vi "Insert Vi by Node.vi"(8 "error in":errorcluster caption="错误输入（无错误）", 9 "dynamic VI*":refnum<vi>, 10 "Node*":refnum<data-value>, 11 "PanelRootNode 输入":refnum<class "PanelRootNode.lvclass"> caption="DNL_LabVIEW Object in") -> (0 "error out":errorcluster caption="错误输出", 3 "PanelRootNode 输出":refnum<class "PanelRootNode.lvclass"> caption="DNL_LabVIEW Object out")   [LabVIEW 2016, in "PanelRootNode.lvclass"]
uses:
  PanelRootNode.lvclass
  C:/Users/CL/Desktop/ZcDAQprj0811/ZcDAQprj/Modules/DAQ-Display/PanelSplitToolkit/PanelLinkNode/PanelLinkNode.lvclass
  PanelObject/PanelObject.lvclass
  PanelLinkNode/PanelLinkNode.lvclass/PanelLinkNode.ctl
  PanelDataNode/PanelDataNode.lvclass
  PanelLinkNode/PanelLinkNode.lvclass
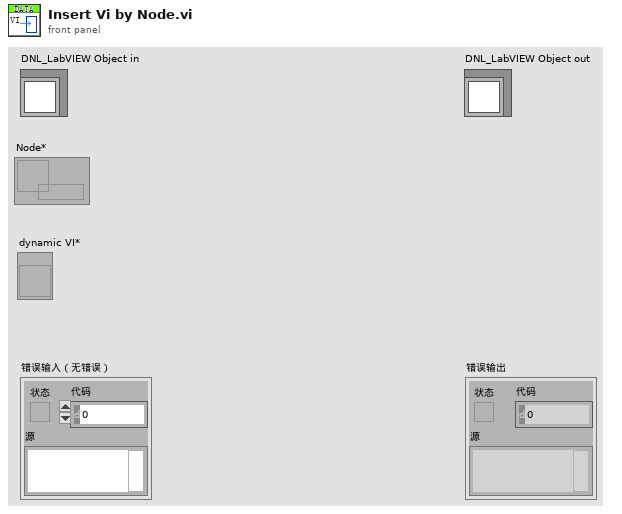
[diagram p1: front panel]
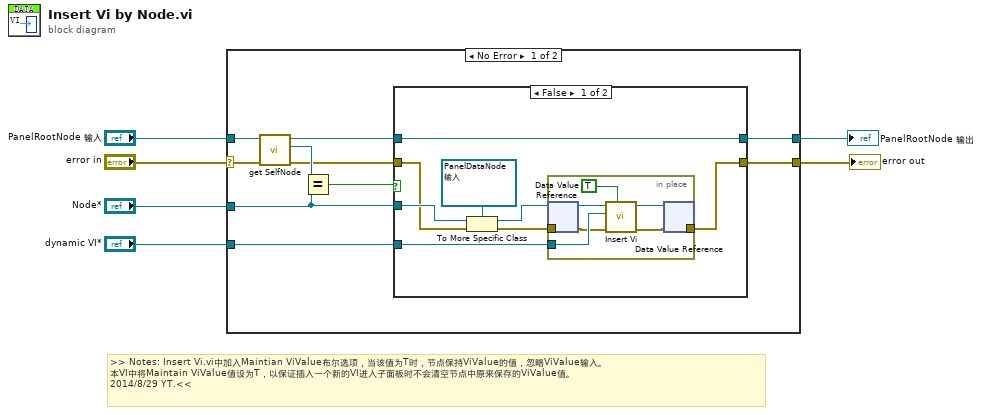
[diagram p0: block diagram]
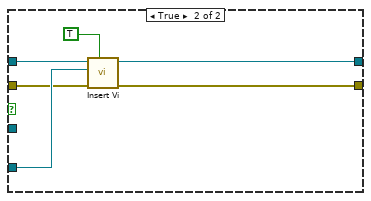
[diagram p2: hidden frame]
diagram:
  # ">> Notes: Insert Vi.vi中加入Maintian ViValue布尔选项，当该值为T时，节点保持ViValue的值，忽略ViValue输入。\n本VI中将Maintain ViValue值设为T，以保证插入一个新的VI进入子面板时不会清空节点中原来保存的ViValue值。\n2014/8/29 YT.<<"
  n1 = case shown="No Error" "error in" {
    selector: "error in" -> [w10 w38]
    tunnel: [w11 w38] -> w5
    tunnel: [w16 w37] -> w3
    tunnel: "PanelRootNode 输入" -> [w15 w37]
    tunnel: "Node*" -> [w13 _]
    tunnel: "dynamic VI*" -> [w8 _]
    frame No Error {
      n2 = call "get SelfNode.vi"("error in (no error)"=w10, "PanelLinkNode输入"=w15) -> ("error out"=w7:errorcluster, "SelfNode*"=w14:refnum<data-value>, "PanelLinkNode输出"=w9:refnum<class "PanelRootNode.lvclass">)  [unwired: 7 in]
      n3 = Equal?(x=w14, y=w13) -> (x = y?=w12:bool)
      n4 = case shown="False" w12 {
        tunnel: w9 -> [w17 w36]
        tunnel: w8 -> [w24 w35]
        tunnel: [w17 w34] -> w16
        tunnel: w7 -> [w19 w33]
        tunnel: w13 -> [w21 _]
        tunnel: [w23 w32] -> w11
        frame False {
          n5 = To More Specific Class(target class=refnum<data-value> refnum ("数据值引用"), reference=w21, error in=w19) -> (specific class reference=w20:refnum<data-value>, error out=w18:errorcluster)
          n6 = in-place {
            in-place-border: w24 -> [w30]
            in-place-border: w18 -> [w27]
            in-place-border: [w26] -> w23
            n7 = in-place-dvr #1(w20) -> (w29:refnum<class "PanelDataNode.lvclass">)  [unwired: 1 out]
            n8 = call-dynamic "Insert Vi.vi"("Maintain ViValue(F)"=TRUE, "error in (no error)"=w27, "VI*"=w30, "PanelDataNode 输入"=w29) -> ("error out"=w26:errorcluster, "PanelDataNode 输出"=w28:refnum<class "PanelDataNode.lvclass">)  [unwired: 6 in]
            n9 = in-place-dvr #1(w28) -> ()  [unwired: 2 out]
          }
        }
        frame True {
          n10 = call-dynamic "Insert Vi.vi"("Maintain ViValue(F)"=TRUE, "error in (no error)"=w33, "VI*"=w35, "PanelDataNode 输入"=w36) -> ("error out"=w32:errorcluster, "PanelDataNode 输出"=w34:refnum<class "PanelRootNode.lvclass">)  [unwired: 6 in]
        }
      }
    }
    frame Error {
    }
  }
  "error out" <- w5
  "PanelRootNode 输出" <- w3
